vi "Temperature Converter.vi"() -> ()   [LabVIEW 2014]
panel:
  in  "stop":bool
  out "Converted Temperature":dbl
  in  "Temperature":dbl
  in  "Enum":T1(ring)
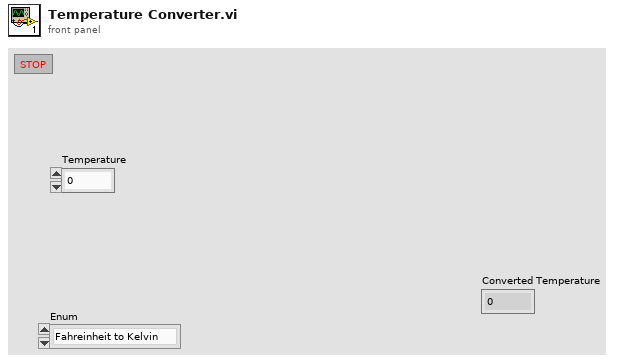
[diagram p1: front panel]
types:
  T1 = enum16{"Fahreinheit to Kelvin", "Celsius to Fahreinheit", "Fahrenheit to Celsius", "Celsius to Kelvin"}
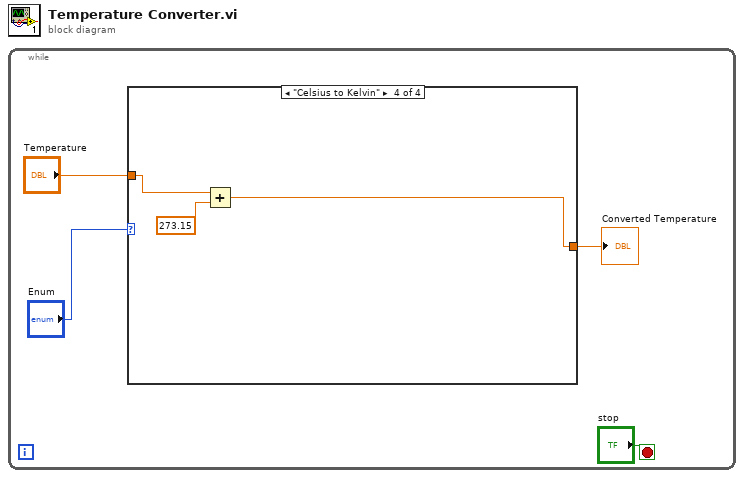
[diagram p0: block diagram]
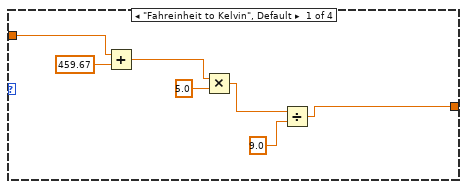
[diagram p2: hidden frame]
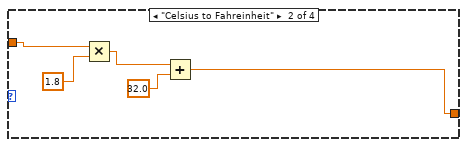
[diagram p3: hidden frame]
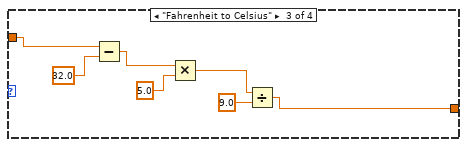
[diagram p4: hidden frame]
diagram:
  n1 = while {
    stop <- "stop" stop-if-true
    n2 = case shown="\"Celsius to Kelvin\"" "Enum" {
      tunnel: "Temperature" -> [w11 w16 w23 w26]
      tunnel: [w5 w12 w17 w24] -> w2
      frame "Fahreinheit to Kelvin", Default {
        n3 = Add(x=w11, y=459.67) -> (x+y=w9:dbl)
        n4 = Multiply(x=w9, y=5.0) -> (x*y=w7:dbl)
        n5 = Divide(x=w7, y=9.0) -> (x/y=w5:dbl)
      }
      frame "Celsius to Fahreinheit" {
        n6 = Multiply(x=w16, y=1.8) -> (x*y=w14:dbl)
        n7 = Add(x=w14, y=32.0) -> (x+y=w12:dbl)
      }
      frame "Fahrenheit to Celsius" {
        n8 = Subtract(x=w23, y=32.0) -> (x-y=w21:dbl)
        n9 = Multiply(x=w21, y=5.0) -> (x*y=w19:dbl)
        n10 = Divide(x=w19, y=9.0) -> (x/y=w17:dbl)
      }
      frame "Celsius to Kelvin" {
        n11 = Add(x=w26, y=273.15) -> (x+y=w24:dbl)
      }
    }
    "Converted Temperature" <- w2
  }
